vi "Confirm.vi"(8 "error in":errorcluster, 10 "CANopen Message":refnum<class "CANopen Response Message.lvclass">, 11 "SDO Manager in":refnum<class "SDO Manager.lvclass">) -> (0 "error out":errorcluster, 3 "SDO Manager out":refnum<class "SDO Manager.lvclass">)   [LabVIEW 2024, in "CANopen Master.lvlib" / "SDO Manager.lvclass"]
uses:
  SDO Manager.lvclass
  SDO Manager.lvclass/SDO Manager.ctl
  CANopen Response/CANopen Response Message.lvclass
  <vilib>/Utility/miscctls.llb/LVMapReplaceAction.ctl
  CANopen Message/CANopen Message.lvclass
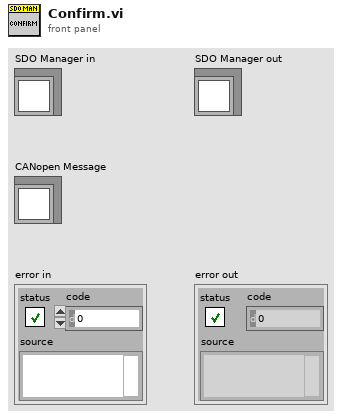
[diagram p1: front panel]
types:
  T1 = typedef "LVMapReplaceAction.ctl" = enum32{"Modify Entry only if found", "Add or Modify Entry", "Delete Entry"}
  T2 = typedef "CANopen Master.lvlib/SDO Manager.lvclass/ObjectAttributes.ctl" = cluster{"SDO Response Map":map{u32, refnum<notifier>}}
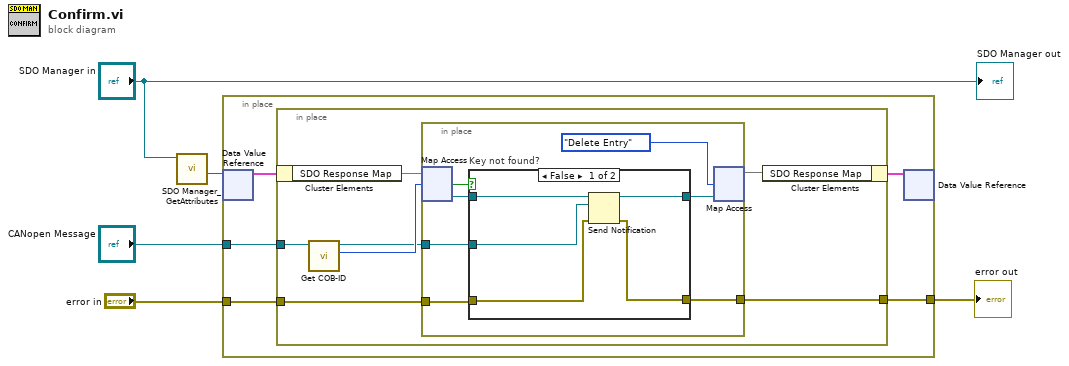
[diagram p0: block diagram]
diagram:
  n1 = call "SDO Manager_GetAttributes.vi"("reference in"="SDO Manager in") -> ("DataRef"=w4:refnum<data-value>)  [unwired: 7 in, 3 out]
  n2 = in-place {
    in-place-border: "error in" -> [w10]
    in-place-border: [w7] -> w2
    in-place-border: "CANopen Message" -> [w6]
    n3 = in-place-dvr #1(w4) -> (w9:T2)  [unwired: 1 out]
    n4 = in-place {
      in-place-border: w10 -> [w17]
      in-place-border: [w14] -> w7
      in-place-border: w6 -> [w13]
      n5 = in-place-cluster #2(w9) -> ("SDO Response Map"=w16:map{u32, refnum<notifier>})
      n6 = call "Get COB-ID.vi"("CANopen Message in"=w13) -> ("COB-ID"=w12:u32, "CANopen Message out"=w11:refnum<class "CANopen Response Message.lvclass">)  [unwired: 9 in]
      n7 = in-place {
        in-place-border: w17 -> [w22]
        in-place-border: [w20] -> w14
        in-place-border: w11 -> [w18]
        n8 = in-place-map #3(w16, w12) -> (w23:refnum<notifier>, w19:bool)  [unwired: 1 in]
        n9 = case "Key not found?" shown="False" w19 {
          tunnel: w23 -> [w29 w31]
          tunnel: w22 -> [w28 w30]
          tunnel: [w27 w31] -> w21
          tunnel: [w26 w30] -> w20
          tunnel: w18 -> [w25 _]
          frame False {
            n10 = Send Notification(notification=w25, notifier=w29, error in (no error)=w28) -> (notifier out=w27:refnum<notifier>, error out=w26:errorcluster)
          }
          frame True {
          }
        }
        n11 = in-place-map #3(w21, LVMapReplaceAction."Delete Entry" ("action")) -> (w15:map{u32, refnum<notifier>})  [unwired: 2 out]
      }
      n12 = in-place-cluster #2("SDO Response Map"=w15) -> (w8:T2)
    }
    n13 = in-place-dvr #1(w8) -> ()  [unwired: 2 out]
  }
  "error out" <- w2
  "SDO Manager out" <- "SDO Manager in"
